vi "Scada_Burglar Project.vi"() -> ()   [LabVIEW 2024]
panel:
  in  "stop":bool
  in  "address 2":string
  in  "Data Input 2":string
  out "IR sensor Value 2":dbl(graph)
  out "Intrusion Detected":bool
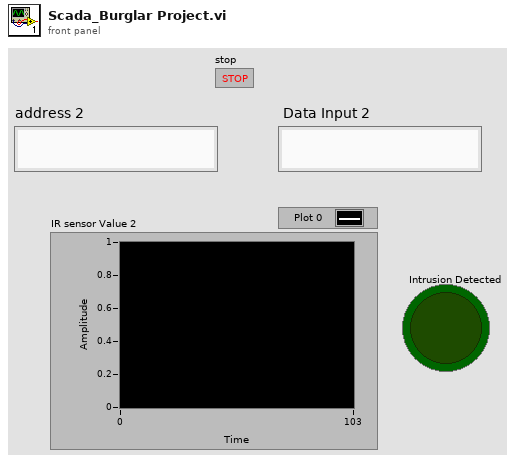
[diagram p1: front panel]
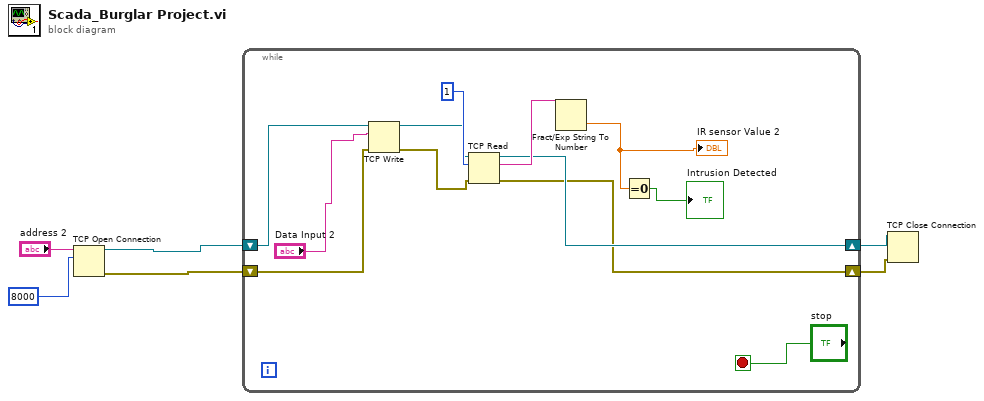
[diagram p0: block diagram]
diagram:
  n1 = TCP Open Connection(address="address 2", remote port or service name=u16 8000) -> (connection ID=w2:refnum<k5>, error out=w1:errorcluster)  [unwired: 3 in]
  n2 = while {
    shift-right: [w14] -> w6
    shift-left: w2 -> [w10]
    shift-right: [w12] -> w5
    shift-left: w1 -> [w9]
    stop <- "stop" stop-if-true
    n3 = TCP Write(connection ID=w10, data in="Data Input 2", error in (no error)=w9) -> (connection ID out=w11:refnum<k5>, error out=w13:errorcluster)  [unwired: 1 in, 1 out]
    n4 = TCP Read(connection ID=w11, bytes to read=1, error in (no error)=w13) -> (connection ID out=w14:refnum<k5>, data out=w17:string, error out=w12:errorcluster)  [unwired: 2 in]
    n5 = Fract/Exp String To Number(string=w17) -> (number=w15:dbl)  [unwired: 3 in, 1 out]
    "IR sensor Value 2" <- w15
    n6 = Equal To 0?(x=w15) -> (x = 0?=→"Intrusion Detected":bool)
  }
  n7 = TCP Close Connection(connection ID=w6, error in (no error)=w5) -> ()  [unwired: 1 in, 2 out]
